vi "GA_Crossover.vi"(6 "Parameters":T1={"Population size"=100, "Generations no."=500, "Crossover probabality"=6.0, "Mutation mode"=enum."one-point, fitness-adjustable rate", "Creep mutation"=FALSE, "Mutation rate"=0.005, "Min mutation rate"=0.005, "Max mutation rate"=0.0005, "Relative fitness differential"=0.25, "Reproduction plan"=enum."Steady-state-replace-random", "Elitism"=FALSE, "FeaturesPerChannel"=0} {"Relative fitness differential" min=0.0 max=1.0; "Max mutation rate" min=0.0 max=1.0; "Min mutation rate" min=0.0 max=1.0; "Mutation rate" min=0.0 max=1.0; "Crossover probabality" min=0.0 max=1.0; "Generations no." min=1; "Population size" min=1}, 10 "Genotype 2":i8[](array[numeric]), 11 "Genotype 1":i8[](array[numeric])) -> (2 "Offspring 2":i8[](array[numeric]), 3 "Offspring 1":i8[](array[numeric]))   [LabVIEW 2016, in "GA.lvlib"]
doc: "Crossovers (mixes) genotypes"
uses:
  GA.lvlib
  GA_tParameters.ctl
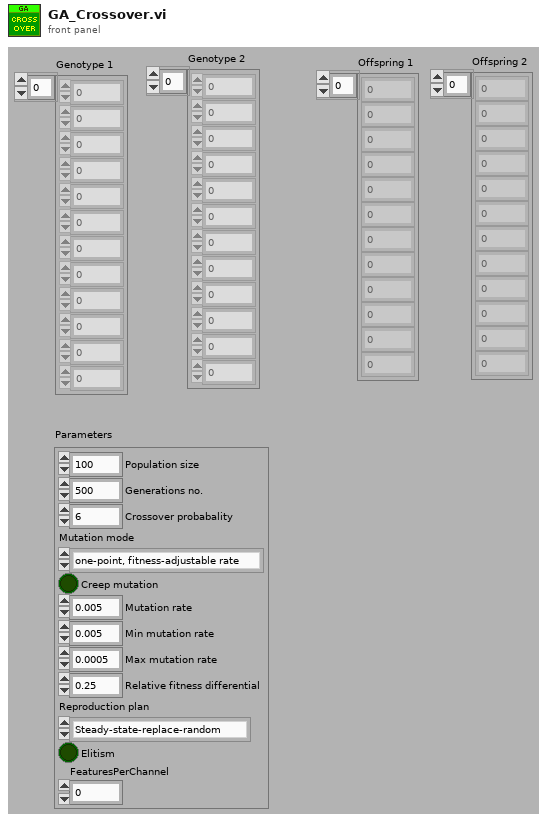
[diagram p1: front panel]
types:
  T1 = typedef "GA.lvlib/GA_tParameters.ctl" = cluster{"Population size":i32, "Generations no.":i32, "Crossover probabality":dbl, "Mutation mode":enum16{"one-point, fixed rate", "one-point, fitness-adjustable rate", "one-point, distance-adjustable rate"}, "Creep mutation":bool, "Mutation rate":dbl, "Min mutation rate":dbl, "Max mutation rate":dbl, "Relative fitness differential":dbl, "Reproduction plan":enum16{"Full generational replacement", "Steady-state-replace-random", "Steady-state-replace-worst"}, "Elitism":bool, "FeaturesPerChannel":i32}
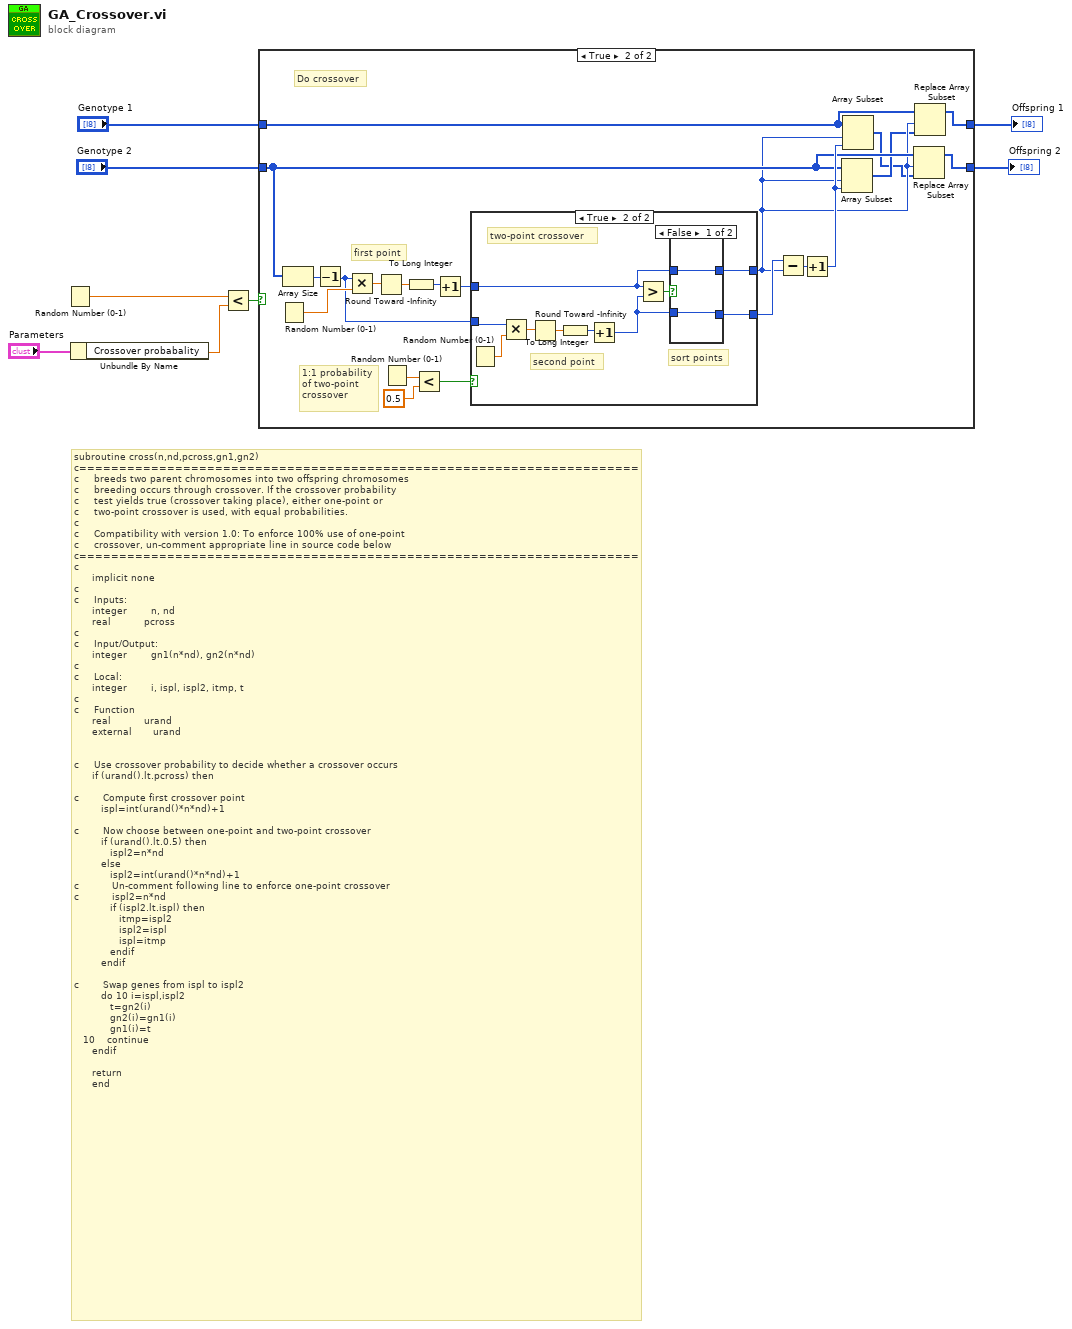
[diagram p0: block diagram]
diagram:
  # "subroutine cross(n,nd,pcross,gn1,gn2)\nc======================================================================\nc     breeds two parent chromosomes into two offspring chromosomes\nc     breeding occurs through crossover. If the crossover probability\nc     test yields true (crossover taking place), either one-point or\nc     two-point crossover is used, with equal probabilities.\nc\nc     Compatibility with version 1.0: To enforce 100% use of one-point\nc     crossover, un-comment appropriate line in source code below\nc======================================================================\nc\n      implicit none\nc\nc     Inputs:\n      integer        n, nd\n      real           pcross\nc\nc     Input/Output:\n      integer        gn1(n*nd), gn2(n*nd)\nc\nc     Local:\n      integer        i, ispl, ispl2, itmp, t\nc\nc     Function\n      real           urand\n      external       urand\n \n \nc     Use crossover probability to decide whether a crossover occurs\n      if (urand().lt.pcross) then\n\nc        Compute first crossover point\n         ispl=int(urand()*n*nd)+1\n \nc        Now choose between one-point and two-point crossover \n         if (urand().lt.0.5) then\n            ispl2=n*nd\n         else\n            ispl2=int(urand()*n*nd)+1\nc           Un-comment following line to enforce one-point crossover\nc           ispl2=n*nd\n            if (ispl2.lt.ispl) then\n               itmp=ispl2\n               ispl2=ispl\n               ispl=itmp\n            endif\n         endif \n \nc        Swap genes from ispl to ispl2\n         do 10 i=ispl,ispl2\n            t=gn2(i)\n            gn2(i)=gn1(i)\n            gn1(i)=t\n   10    continue\n      endif\n \n      return\n      end"
  n1 = Random Number (0-1)() -> (number: 0 to 1=w8:dbl)
  n2 = Unbundle By Name("Parameters") -> ("Crossover probabality"=w1:dbl)
  n3 = Less?(x=w8, y=w1) -> (x < y?=w7:bool)
  n4 = case shown="True" w7 {
    tunnel: [w10 w13] -> w4
    tunnel: "Genotype 1" -> [w10 w17]
    tunnel: [w9 w14] -> w3
    tunnel: "Genotype 2" -> [w9 w16]
    frame False {
      # "no crossover"
    }
    frame True {
      # "1:1 probability\nof two-point\ncrossover"
      # "Do crossover"
      # "first point"
      n5 = Random Number (0-1)() -> (number: 0 to 1=w26:dbl)
      n6 = Array Size(array=w16) -> (size(s)=w27:i32)
      n7 = Decrement(x=w27) -> (x-1=w21:i32)
      n8 = Multiply(x=w21, y=w26) -> (x*y=w25:dbl)
      n9 = Round Toward -Infinity(1:w25) -> (0:w24:dbl)
      n10 = Random Number (0-1)() -> (number: 0 to 1=w30:dbl)
      n11 = To Long Integer(number=w24) -> (32bit integer=w23:i32)
      n12 = Less?(x=w30, y=0.5) -> (x < y?=w28:bool)
      n13 = Increment(x=w23) -> (x+1=w22:i32)
      n14 = case shown="True" w28 {
        tunnel: w22 -> [w32 w36]
        tunnel: w21 -> [w31 w39]
        tunnel: [w32 w34] -> w15
        tunnel: [w31 w33] -> w20
        frame False {
          # "one-point crossover"
        }
        frame True {
          # "sort points"
          # "two-point crossover"
          # "second point"
          n15 = Random Number (0-1)() -> (number: 0 to 1=w38:dbl)
          n16 = Multiply(x=w39, y=w38) -> (x*y=w40:dbl)
          n17 = Round Toward -Infinity(1:w40) -> (0:w41:dbl)
          n18 = To Long Integer(number=w41) -> (32bit integer=w42:i32)
          n19 = Increment(x=w42) -> (x+1=w35:i32)
          n20 = Greater?(x=w36, y=w35) -> (0:w37:bool)
          n21 = case shown="False" w37 {
            tunnel: w36 -> [w44 w46]
            tunnel: w35 -> [w43 w45]
            tunnel: [w43 w46] -> w33
            tunnel: [w44 w45] -> w34
            frame False {
            }
            frame True {
            }
          }
        }
      }
      n22 = Subtract(x=w20, y=w15) -> (x-y=w19:i32)
      n23 = Increment(x=w19) -> (x+1=w18:i32)
      n24 = Array Subset(array=w16, index=w15, length=w18) -> (w12:i8[])
      n25 = Array Subset(array=w17, index=w15, length=w18) -> (w11:i8[])
      n26 = Replace Array Subset(array=w16, new element=w11, index=w15) -> (w14:i8[])
      n27 = Replace Array Subset(array=w17, new element=w12, index=w15) -> (w13:i8[])
    }
  }
  "Offspring 1" <- w4
  "Offspring 2" <- w3
